vi "Initialization VI.vi"(8 "error in (no error)":errorcluster, 10 "Custom XML":string, 11 "Device Item Ref in":T1 format="%.0x") -> (0 "error out":errorcluster, 3 "Device Item Ref out":T1 format="%.0x")   [LabVIEW 2020, in "FlexRay Custom Device System Explorer.lvlib"]
uses:
  FlexRay Custom Device System Explorer.lvlib
  <vilib>/NI VeriStand/Custom Device API/Custom Device Item Ref.ctl
  <vilib>/NI VeriStand/Custom Device API/Custom Device Channel.ctl
  <vilib>/NI VeriStand/Custom Device API/Custom Device Channel Type.ctl
  Shared/Constants.vi
  <vilib>/NI VeriStand/Custom Device API/Custom Device API.lvlib
  Shared/FlexRay Custom Device Shared.lvlib
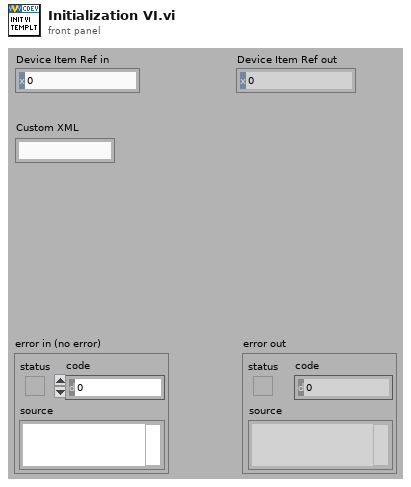
[diagram p1: front panel]
types:
  T1 = typedef "Custom Device API.lvlib/Custom Device Item Ref.ctl" = u64
  T2 = typedef "Custom Device API.lvlib/Custom Device Channel.ctl" = cluster{"Type":T3, "Units":string, "Default Value":dbl, "Faultable":bool, "Scalable":bool}
  T3 = typedef "Custom Device API.lvlib/Custom Device Channel Type.ctl" = enum16{"Input", "Output"}
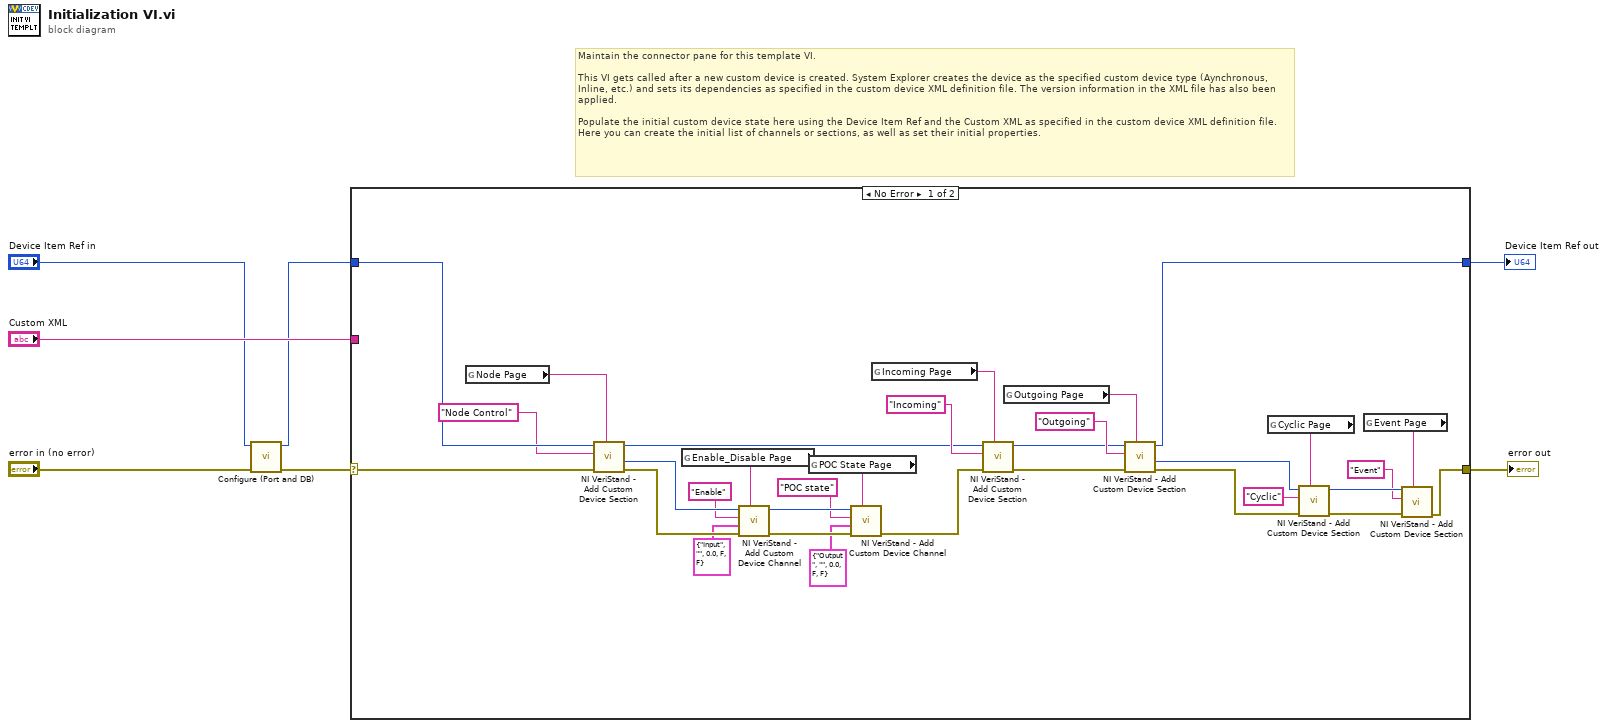
[diagram p0: block diagram]
diagram:
  # "Maintain the connector pane for this template VI.\n\nThis VI gets called after a new custom device is created. System Explorer creates the device as the specified custom device type (Aynchronous, Inline, etc.) and sets its dependencies as specified in the custom device XML definition file. The version information in the XML file has also been applied.\n\nPopulate the initial custom device state here using the Device Item Ref and the Custom XML as specified in the custom device XML definition file. Here you can create the initial list of channels or sections, as well as set their initial properties."
  n1 = call "Configure (Port and DB).vi"("error in (no error)"="error in (no error)", "Device Item Ref in"="Device Item Ref in") -> ("error out"=w3:errorcluster, "Device Item Ref out"=w1:T1)  [unwired: 8 in]
  n2 = case shown="No Error" w3 {
    selector: w3 -> [w23 w41]
    tunnel: [w29 w41] -> w7
    tunnel: [w36 w40] -> w6
    tunnel: w1 -> [w22 w40]
    tunnel: "Custom XML" -> [_ _]
    frame No Error {
      n3 = global read "Constants.vi" "Node Page"() -> (w15:string)
      n4 = call <vilib>:"NI VeriStand - Add Custom Device Section.vi"("GUID (Default Section)"=w15, "error in (no error)"=w23, "Section Name"="Node Control", "Parent Ref in"=w22) -> ("error out"=w18:errorcluster, "Section Ptr"=w19:T1, "Parent Ref out"=w21:T1)  [unwired: 4 in, 1 out]
      n5 = global read "Constants.vi" "Enable_Disable Page"() -> (w14:string)
      n6 = call <vilib>:"NI VeriStand - Add Custom Device Channel.vi"("GUID (Default Channel)"=w14, "error in (no error)"=w18, "Channel"=T2 {"Type"=enum."Input", "Units"="", "Default Value"=0.0, "Faultable"=FALSE, "Scalable"=FALSE}, "Channel Name"="Enable", "Parent Ref in"=w19) -> ("error out"=w12:errorcluster, "Parent Ref out"=w11:T1)  [unwired: 3 in, 2 out]
      n7 = global read "Constants.vi" "POC State Page"() -> (w8:string)
      n8 = call <vilib>:"NI VeriStand - Add Custom Device Channel.vi"("GUID (Default Channel)"=w8, "error in (no error)"=w12, "Channel"=T2 {"Type"=enum."Output", "Units"="", "Default Value"=0.0, "Faultable"=FALSE, "Scalable"=FALSE}, "Channel Name"="POC state", "Parent Ref in"=w11) -> ("error out"=w13:errorcluster)  [unwired: 3 in, 3 out]
      n9 = global read "Constants.vi" "Incoming Page"() -> (w26:string)
      n10 = call <vilib>:"NI VeriStand - Add Custom Device Section.vi"("GUID (Default Section)"=w26, "error in (no error)"=w13, "Section Name"="Incoming", "Parent Ref in"=w21) -> ("error out"=w24:errorcluster, "Parent Ref out"=w37:T1)  [unwired: 4 in, 2 out]
      n11 = global read "Constants.vi" "Outgoing Page"() -> (w25:string)
      n12 = call <vilib>:"NI VeriStand - Add Custom Device Section.vi"("GUID (Default Section)"=w25, "error in (no error)"=w24, "Section Name"="Outgoing", "Parent Ref in"=w37) -> ("error out"=w34:errorcluster, "Section Ptr"=w35:T1, "Parent Ref out"=w36:T1)  [unwired: 4 in, 1 out]
      n13 = global read "Constants.vi" "Cyclic Page"() -> (w28:string)
      n14 = call <vilib>:"NI VeriStand - Add Custom Device Section.vi"("GUID (Default Section)"=w28, "error in (no error)"=w34, "Section Name"="Cyclic", "Parent Ref in"=w35) -> ("error out"=w32:errorcluster, "Parent Ref out"=w31:T1)  [unwired: 4 in, 2 out]
      n15 = global read "Constants.vi" "Event Page"() -> (w27:string)
      n16 = call <vilib>:"NI VeriStand - Add Custom Device Section.vi"("GUID (Default Section)"=w27, "error in (no error)"=w32, "Section Name"="Event", "Parent Ref in"=w31) -> ("error out"=w29:errorcluster)  [unwired: 4 in, 3 out]
    }
    frame Error {
    }
  }
  "error out" <- w7
  "Device Item Ref out" <- w6
